vi "Ave COUNT Query.vi"(8 "error in (no error)":errorcluster, 11 "VISA resource name":refnum<visa-resource-name>) -> (0 "error out":errorcluster, 2 "Measurement":dbl, 3 "VISA resource name out":refnum<visa-resource-name>)   [LabVIEW 2017, in "ADCMT7451_ADC.lvlib"]
doc: "Queries the result of Max/Min calculation."
uses:
  ADCMT7451_ADC.lvlib
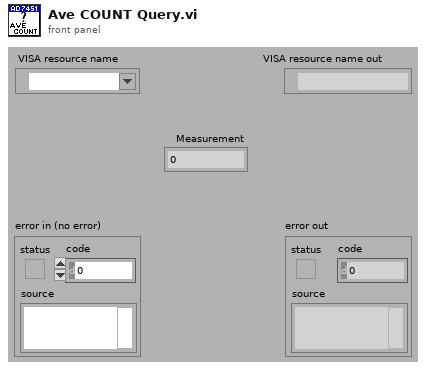
[diagram p1: front panel]
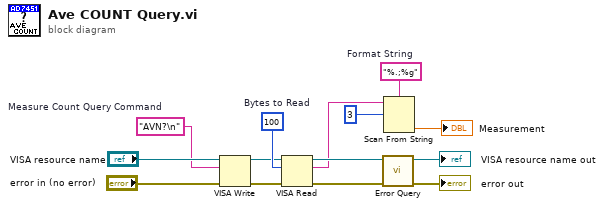
[diagram p0: block diagram]
diagram:
  w5 = "%.;%g"  # Format String
  w2 = "AVN?\n"  # Measure Count Query Command
  w13 = u32 100  # Bytes to Read
  n1 = VISA Write(VISA resource name="VISA resource name", write buffer=w2, error in (no error)="error in (no error)") -> (VISA resource name out=w12:refnum<visa-resource-name>, error out=w11:errorcluster)  [unwired: 1 out]
  n2 = VISA Read(VISA resource name=w12, byte count=w13, error in (no error)=w11) -> (VISA resource name out=w9:refnum<visa-resource-name>, read buffer=w3:string, error out=w10:errorcluster)  [unwired: 1 out]
  n3 = call "Error Query.vi"("error in (no error)"=w10, "VISA resource name"=w9) -> ("error out"=→"error out":errorcluster, "VISA resource name out"=→"VISA resource name out":refnum<visa-resource-name>)  [unwired: 6 in, 2 out]
  n4 = Scan From String(format string=w5, input string=w3, initial scan location=3) -> (output 1=→"Measurement":dbl)  [unwired: 2 in, 3 out]
